vi "Obtain all split file speed data file paths.vi"(11 "Speed data file path & name (any)":path) -> (1 "Number of speed data split files (= number of trials)":i32, 3 "Trial speed data split file paths":path[](array[path]))   [LabVIEW 2020]
uses:
  <userlib>/_OpenG.lib/array/array.llb/Conditional Auto-Indexing Tunnel (Path)__ogtk.vi
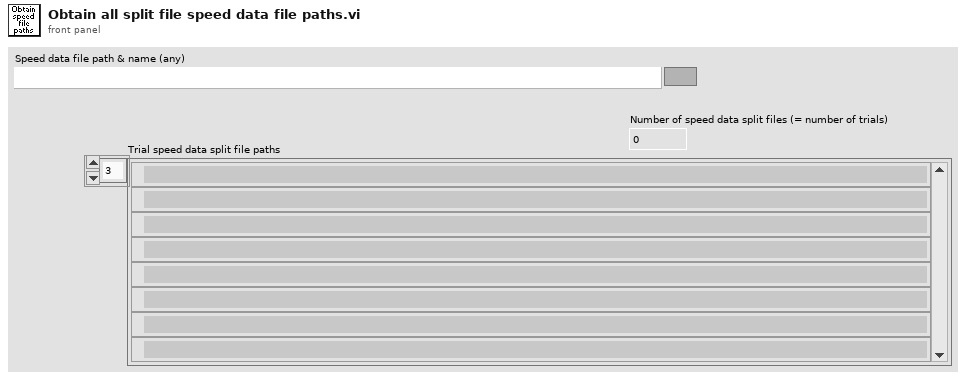
[diagram p1: front panel]
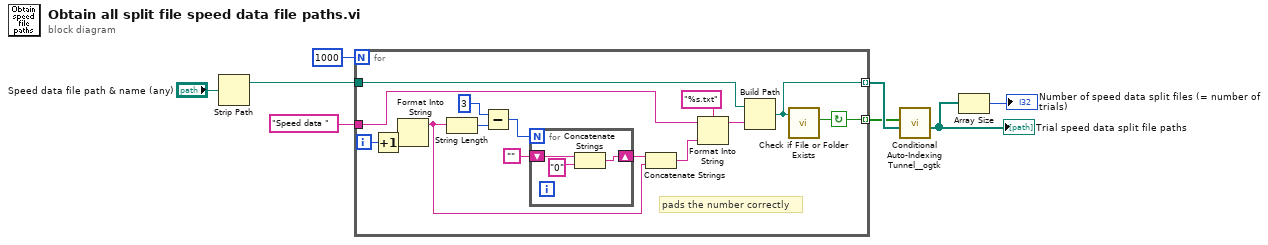
[diagram p0: block diagram]
diagram:
  n1 = Strip Path(path="Speed data file path & name (any)") -> (stripped path=w4:path)  [unwired: 1 out]
  n2 = for {
    N: 1000 -> [_]
    tunnel: w4 -> [w12]
    tunnel: "Speed data " ("Pad Character (\\s)") -> [w14]
    tunnel: [w13] -> w7 mode=indexing
    tunnel: [w11] -> w8 mode=indexing
    i -> [w23]
    stop <- w13 continue-if-true
    # "pads the number correctly"
    n3 = Increment(x=w23) -> (x+1=w10:i32)
    n4 = Format Into String(w10) -> (resulting string=w17:string)  [unwired: 3 in, 1 out]
    n5 = String Length(string=w17) -> (length=w21:i32)
    n6 = Subtract(x=3 ("End Length"), y=w21) -> (x-y=w20:i32)
    n7 = for {
      N: w20 -> [_]
      shift-right: [w24] -> w18
      shift-left: "" ("Pad Character (\\s)") -> [w25]
      n8 = Concatenate Strings(w25, "0" ("Pad Character (\\s)")) -> (w24:string)
    }
    n9 = Concatenate Strings(w18, w17) -> (w16:string)
    n10 = Format Into String(format string="%s.txt", initial string=w14, w16) -> (resulting string=w15:string)  [unwired: 1 in, 1 out]
    n11 = Build Path(base path=w12, name or relative path=w15) -> (appended path=w11:path)
    n12 = call <vilib>:"Check if File or Folder Exists.vi"("path"=w11) -> ("file or folder exists?"=w13:bool)  [unwired: 8 in, 2 out]
  }
  n13 = call-poly <userlib>:"Conditional Auto-Indexing Tunnel__ogtk.vi"("Array in"=w8, "Elements to keep"=w7) -> ("Filtered Array out"=w2:path[])  [unwired: 5 in]
  "Trial speed data split file paths" <- w2
  n14 = Array Size(array=w2) -> (size(s)=→"Number of speed data split files (= number of trials)":i32)
